vi "buffer test 0.3-7.1.vi"() -> (4 "[X,R]":dbl=7.720664e-07, 6 "[Y,0]":dbl=-91.958315)   [LabVIEW 2010]
panel:
  out "Waveform Chart":dbl(graph)
  in  "830 GPIB 8":string="8"
  in  "Ring":u16(ring) items=["256", "512", "1024", "2048", "4096", "8192", "16384"]
  out "number of points":string="2\r"
  out "Scan over":bool
  in  "ring down time":dbl
  in  "ring time":dbl=3.0
  out "Scan starts":bool
  in  "Sensitivity 3":u16(ring)=12 items=["2nV", "5nV", "10nV", "20nV", "50nV", "100nV", "200nV", "500nV", "1uV", "2uV", "5uV", "10uV", "20uV", "50uV", "100uV", "200uV", "500uV", "1mV", "2mV", "5mV", "10mV", "20mV", "50mV", "100mV", "200mV", "500mV", "1V"]
  in  "Time constant 3":u16(ring)=6 items=["10us", "30us", "100us", "300us", "1ms", "3ms", "10ms", "30ms", "100ms", "300ms", "1s", "3s", "10s"]
  in  "Backslash (\\) codes":string="\n"
  in  "Sampling Rate":u16(ring)=13 items=["62.5 mHz", "125 mHz", "250 mHz", "500 mHz", "1 Hz", "2 Hz", "4 Hz", "8 Hz", "16 Hz", "32 Hz", "64 Hz, 256 s wait", "128 Hz, 128 s wait", "256 Hz, 64 s wait", "512 Hz, 32 s wait"]
  in  "Data Select":u16(ring)=1 items=["X and Y", "R and Theta"]
  in  "Resonance  Frequency":dbl=486.9
  in  "?":dbl(ring) items=["(kHz)", "(Hz)"]
  in  "freq shift(Hz)":dbl
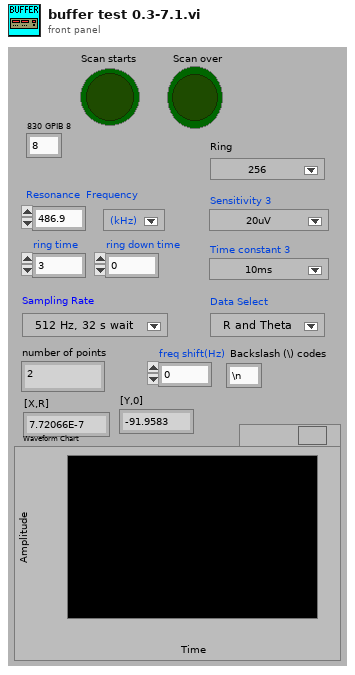
[diagram p1: front panel]
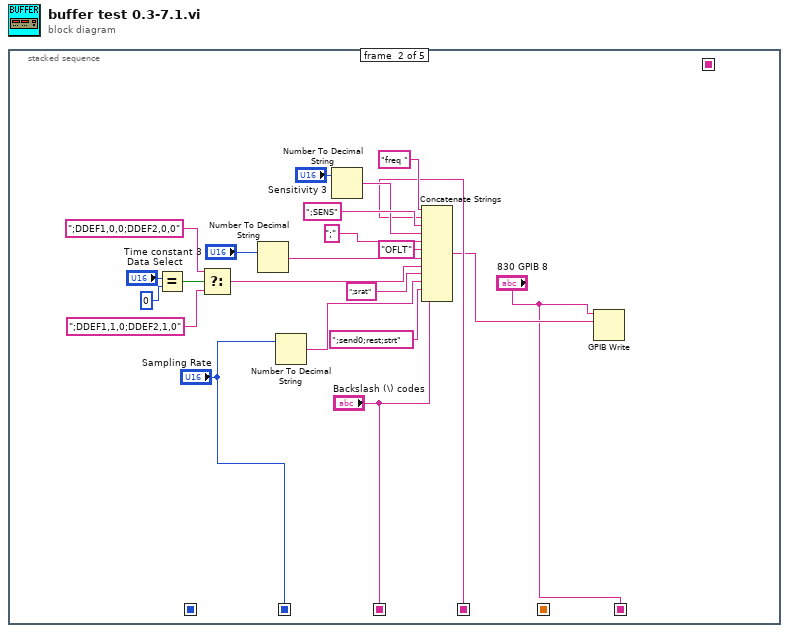
[diagram p0: block diagram]
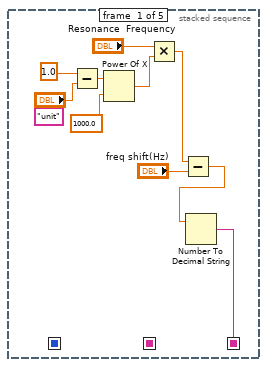
[diagram p2: hidden frame]
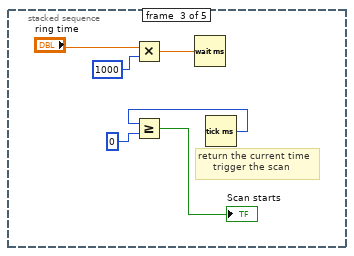
[diagram p3: hidden frame]
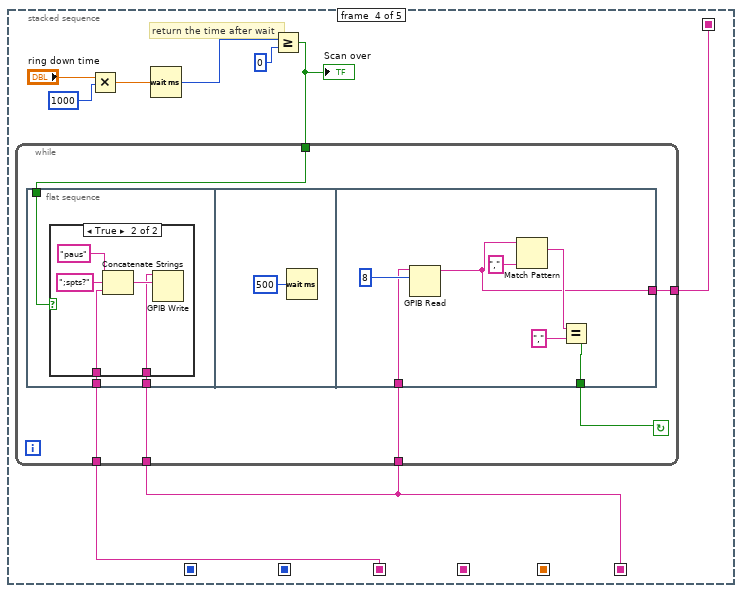
[diagram p4: hidden frame]
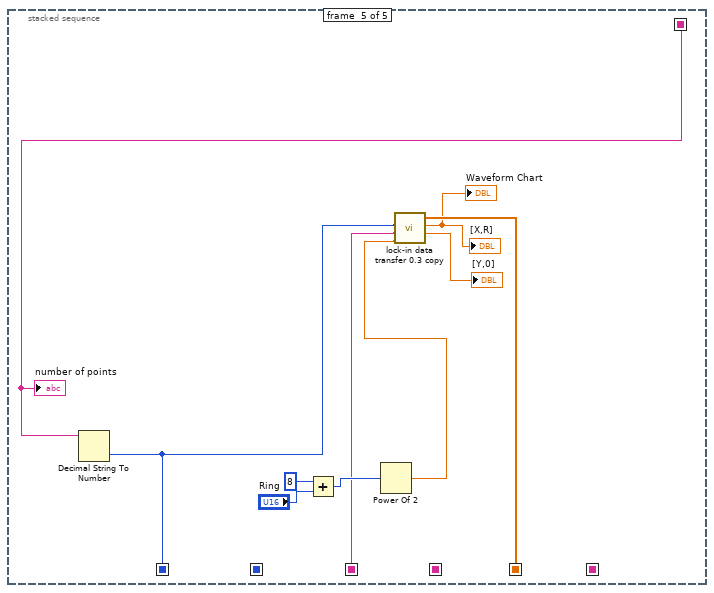
[diagram p6: hidden frame]
diagram:
  n1 = stacked-sequence {
    seq-local: [_ _ _ _ w75] -> [_ _ _ _ _]
    seq-local: [_ "Sampling Rate" _ _ _] -> [_ _ _ _ _]
    seq-local: [_ "830 GPIB 8" _ _ _] -> [_ _ _ w40 _]
    seq-local: [w1 _ _ _ _] -> [_ w21 _ _ _]
    seq-local: [_ _ _ _ w71] -> [_ _ _ _ _]
    seq-local: [_ "Backslash (\\) codes" _ _ _] -> [_ _ _ w45 w72]
    seq-local: [_ _ _ w39 _] -> [_ _ _ _ w76]
    frame #0 {
      (unwired) "unit"
      n2 = Subtract(x=1.0, y="?") -> (x-y=w7:dbl)
      n3 = Power Of X(1:1000.0 ("x"), 2:w7) -> (0:w5:dbl)
      n4 = Multiply(x="Resonance  Frequency", y=w5) -> (x*y=w4:dbl)
      n5 = Subtract(x=w4, y="freq shift(Hz)") -> (x-y=w2:dbl)
      n6 = Number To Decimal String(number=w2) -> (decimal integer string=w1:string)  [unwired: 1 out]
    }
    frame #1 {
      n7 = Equal?(x="Data Select", y=u16 0) -> (x = y?=w14:bool)
      n8 = Select(t=";DDEF1,0,0;DDEF2,0,0" ("string"), s=w14, f=";DDEF1,1,0;DDEF2,1,0" ("string")) -> (s? t:f=w13:string)
      n9 = Number To Decimal String(number="Time constant 3") -> (decimal integer string=w26:string)  [unwired: 1 out]
      n10 = Number To Decimal String(number="Sampling Rate") -> (decimal integer string=w25:string)  [unwired: 1 out]
      n11 = Number To Decimal String(number="Sensitivity 3") -> (decimal integer string=w29:string)  [unwired: 1 out]
      n12 = Concatenate Strings("freq " ("string"), w21, ";SENS", w29, ";" ("string"), "OFLT" ("string"), w26, w13, ";srat" ("string"), w25, ";send0;rest;strt", "Backslash (\\) codes") -> (w12:string)
      n13 = GPIB Write(0:"830 GPIB 8", 1:w12) -> ()  [unwired: 1 in, 4 out]
    }
    frame #2 {
      # "return the current time\n     trigger the scan"
      n14 = Multiply(x="ring time", y=1000) -> (x*y=w38:dbl)
      n15 = Wait (ms)(milliseconds to wait=w38) -> ()  [unwired: 1 out]
      n16 = Tick Count (ms)() -> (millisecond timer value=w34:u32)
      n17 = Greater Or Equal?(x=w34, y=0) -> (x >= y?=→"Scan starts":bool)
    }
    frame #3 {
      # "return the time after wait"
      n18 = Multiply(x="ring down time", y=1000) -> (x*y=w46:dbl)
      n19 = Wait (ms)(milliseconds to wait=w46) -> (millisecond timer value=w44:u32)
      n20 = Greater Or Equal?(x=w44, y=u32 0) -> (x >= y?=w42:bool)
      "Scan over" <- w42
      n21 = while {
        tunnel: w45 -> [w53]
        tunnel: w42 -> [w52]
        tunnel: w40 -> [w50]
        tunnel: w40 -> [w49]
        tunnel: [w48] -> w39
        stop <- w51 continue-if-true
        n22 = flat-sequence {
          tunnel: w53 -> [w56]
          tunnel: w52 -> [w55]
          tunnel: w49 -> [w54]
          tunnel: [w69] -> w51
          tunnel: w50 -> [w64]
          tunnel: [w63] -> w48
          frame #0 {
            n23 = case shown="True" w55 {
              tunnel: w56 -> [_ w59]
              tunnel: w54 -> [_ w57]
              frame False {
              }
              frame True {
                n24 = Concatenate Strings("paus" ("string"), ";spts?" ("string"), w59) -> (w60:string)
                n25 = GPIB Write(0:w57, 1:w60) -> ()  [unwired: 1 in, 4 out]
              }
            }
          }
          frame #1 {
            n26 = Wait (ms)(milliseconds to wait=u32 500) -> ()  [unwired: 1 out]
          }
          frame #2 {
            n27 = GPIB Read(0:w64, 1:8) -> (5:w63:string)  [unwired: 1 in, 4 out]
            n28 = Match Pattern(string=w63, regular expression=",") -> (match substring=w67:string)  [unwired: 4 out]
            n29 = Equal?(x=w67, y="," ("regular expression")) -> (x = y?=w69:bool)
          }
        }
      }
    }
    frame #4 {
      n30 = Decimal String To Number(string=w76) -> (number=w71:i32)  [unwired: 3 out]
      n31 = Add(x=u16 8, y="Ring") -> (x+y=w77:u16)
      n32 = Power Of 2(x=w77) -> (2^x=w73:dbl)
      n33 = call "lock-in data transfer 0.3 copy.vi"("points in buffer"=w73, "string"=w72, "number of points"=w71) -> ("Average\n[Y.0]"=→"[Y,0]":dbl, "Average\n[X, R]"=→"[X,R]" →"Waveform Chart":dbl, "Array x"=w75:dbl[])  [unwired: 2 out]
      "number of points" <- w76
    }
  }
